vi "timeStampSGP4.vi"() -> (0 "Minutes since epoch 1jan 1950":dbl)   [LabVIEW 2015]
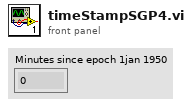
[diagram p1: front panel]
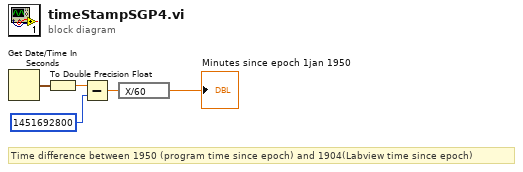
[diagram p0: block diagram]
diagram:
  # "Time difference between 1950 (program time since epoch) and 1904(Labview time since epoch)"
  n1 = Get Date/Time In Seconds() -> (seconds since 1Jan1904=w4:timestamp)
  n2 = To Double Precision Float(number=w4) -> (double precision float=w3:dbl)
  n3 = Subtract(x=w3, y=1451692800) -> (x-y=w2:dbl)
  n4 = expression code="X/60"(w2) -> (→"Minutes since epoch 1jan 1950":dbl)
